vi "Teleop.vi"(10 "Match Info":T1={"Autonomous Elapsed Seconds"=0.0, "TeleOp Elapsed Seconds"=0.0, "Disabled Elapsed Seconds"=0.0, "Visited Autonomous"=FALSE, "Visited TeleOp"=FALSE, "Visited Disabled"=FALSE, "Autonomous Settings"={"Autonomous Style"=enum."Independent", "VI Refnum"=refnum}}, 11 "Call Context":T2) -> ()   [LabVIEW 2019]
doc: "This VI is called for each TeleOp packet received from the DS where the robot is not disabled. It is often used to read from the joysticks and update I/O or to update setpoints for timed control loops. It should complete and return within 20 milliseconds or it may miss DS packets."
uses:
  <vilib>/Rock Robotics/WPI/DriverStation/WPI_DriverStationDerivedRobotMode.ctl
  <vilib>/Rock Robotics/WPI/DriverStation/WPI_DriverStationMatch Info.ctl
  <vilib>/Rock Robotics/WPI/Utilities/WPI_GetSetVariantRefNum.vi
  <vilib>/Rock Robotics/Network Tables/NT Write Numeric Array.vi
  <vilib>/Rock Robotics/Network Tables/NT Read Boolean.vi
  <vilib>/Rock Robotics/Network Tables/NT Read Number.vi
  <vilib>/Rock Robotics/Network Tables/NT Write Boolean Array.vi
panel:
  in  "45 % DC":bool
  in  "35 % DC":bool
  in  "25 % DC":bool
  out "Sample Slider 0":dbl(slide) scale=0.0..5.0
  out "Sample Boolean 1":bool
  out "Sample Boolean 0":bool
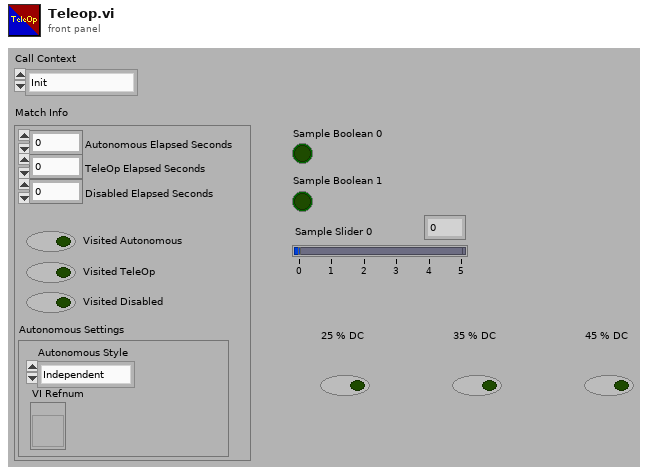
[diagram p1: front panel]
types:
  T1 = typedef "WPI_DriverStationMatch Info.ctl" = cluster{"Autonomous Elapsed Seconds":dbl, "TeleOp Elapsed Seconds":dbl, "Disabled Elapsed Seconds":dbl, "Visited Autonomous":bool, "Visited TeleOp":bool, "Visited Disabled":bool, "Autonomous Settings":cluster{"Autonomous Style":enum16{"Iterative", "Independent"}, "VI Refnum":refnum<vi>}}
  T2 = typedef "WPI_DriverStationDerivedRobotMode.ctl" = enum16{"Init", "Execute", "Stop"}
  T3 = typedef "WPI_JoystickDevRef.ctl" = cluster{"Device":T4}
  T4 = typedef "WPI_JoystickDeviceEnum.ctl" = enum16{"USB 0", "USB 1", "USB 2", "USB 3", "USB 4", "USB 5"}
  T5 = typedef "WPI_RobotDriveDevRef.ctl" = cluster{"DevStatus":errorcluster, "Motors[]":T6[], "Square Inputs":bool, "Max Output":dbl}
  T6 = typedef "WPI_MotorControlDeviceRef.ctl" = cluster{"DeviceStatus":errorcluster, "Type":T7, "PWM":cluster{"PWM Channel":T8, "DeadBand":T9}, "CAN":cluster{"Device Number":u8, "SetOutput VI Ref":variant, "GetOutput VI Ref":variant, "Enable VI Ref":variant, "Disable VI Ref":variant, "Data":variant}, "Invert":bool, "DIO PWM":cluster{"PWM \"Enable\" Channel":T8, "DIOChannel":T10, "PWM Rate":dbl}}
  T7 = typedef "WPI_MotorControlType.ctl" = enum16{"PWM", "CAN", "DIO PWM"}
  T8 = typedef "FPGA_DIOPWMChannel.ctl" = enum8{"PWM 0", "PWM 1", "PWM 2", "PWM 3", "PWM 4", "PWM 5", "PWM 6", "PWM 7", "PWM 8", "PWM 9", "PWM MXP 0", "PWM MXP 1", "PWM MXP 2", "PWM MXP 3", "PWM MXP 4", "PWM MXP 5", "PWM MXP 6", "PWM MXP 7", "PWM MXP 8", "PWM MXP 9", "Invalid"}
  T9 = typedef "WPI_PWMDeadband.ctl" = cluster{"Name":string, "maxPositivePwm":i32, "minPositivePwm":i32, "centerPwm":i32, "maxNegativePwm":i32, "minNegativePwm":i32, "angularRange":u16}
  T10 = typedef "FPGA_DIOChannel.ctl" = enum8{"DIO 0", "DIO 1", "DIO 2", "DIO 3", "DIO 4", "DIO 5", "DIO 6", "DIO 7", "DIO 8", "DIO 9", "DIO MXP 0", "DIO MXP 1", "DIO MXP 2", "DIO MXP 3", "DIO MXP 4", "DIO MXP 5", "DIO MXP 6", "DIO MXP 7", "DIO MXP 8", "DIO MXP 9", "DIO MXP 10", "DIO MXP 11", "DIO MXP 12", "DIO MXP 13", "DIO MXP 14", "DIO MXP 15", "SPI Port CS1", "SPI Port CS2", "SPI Port CS3", "SPI Port MISO", "SPI Port MOSI", "Invalid"}
  T11 = cluster{"JoystickDevRef":T3, "RobotDriveDevRef":T5}
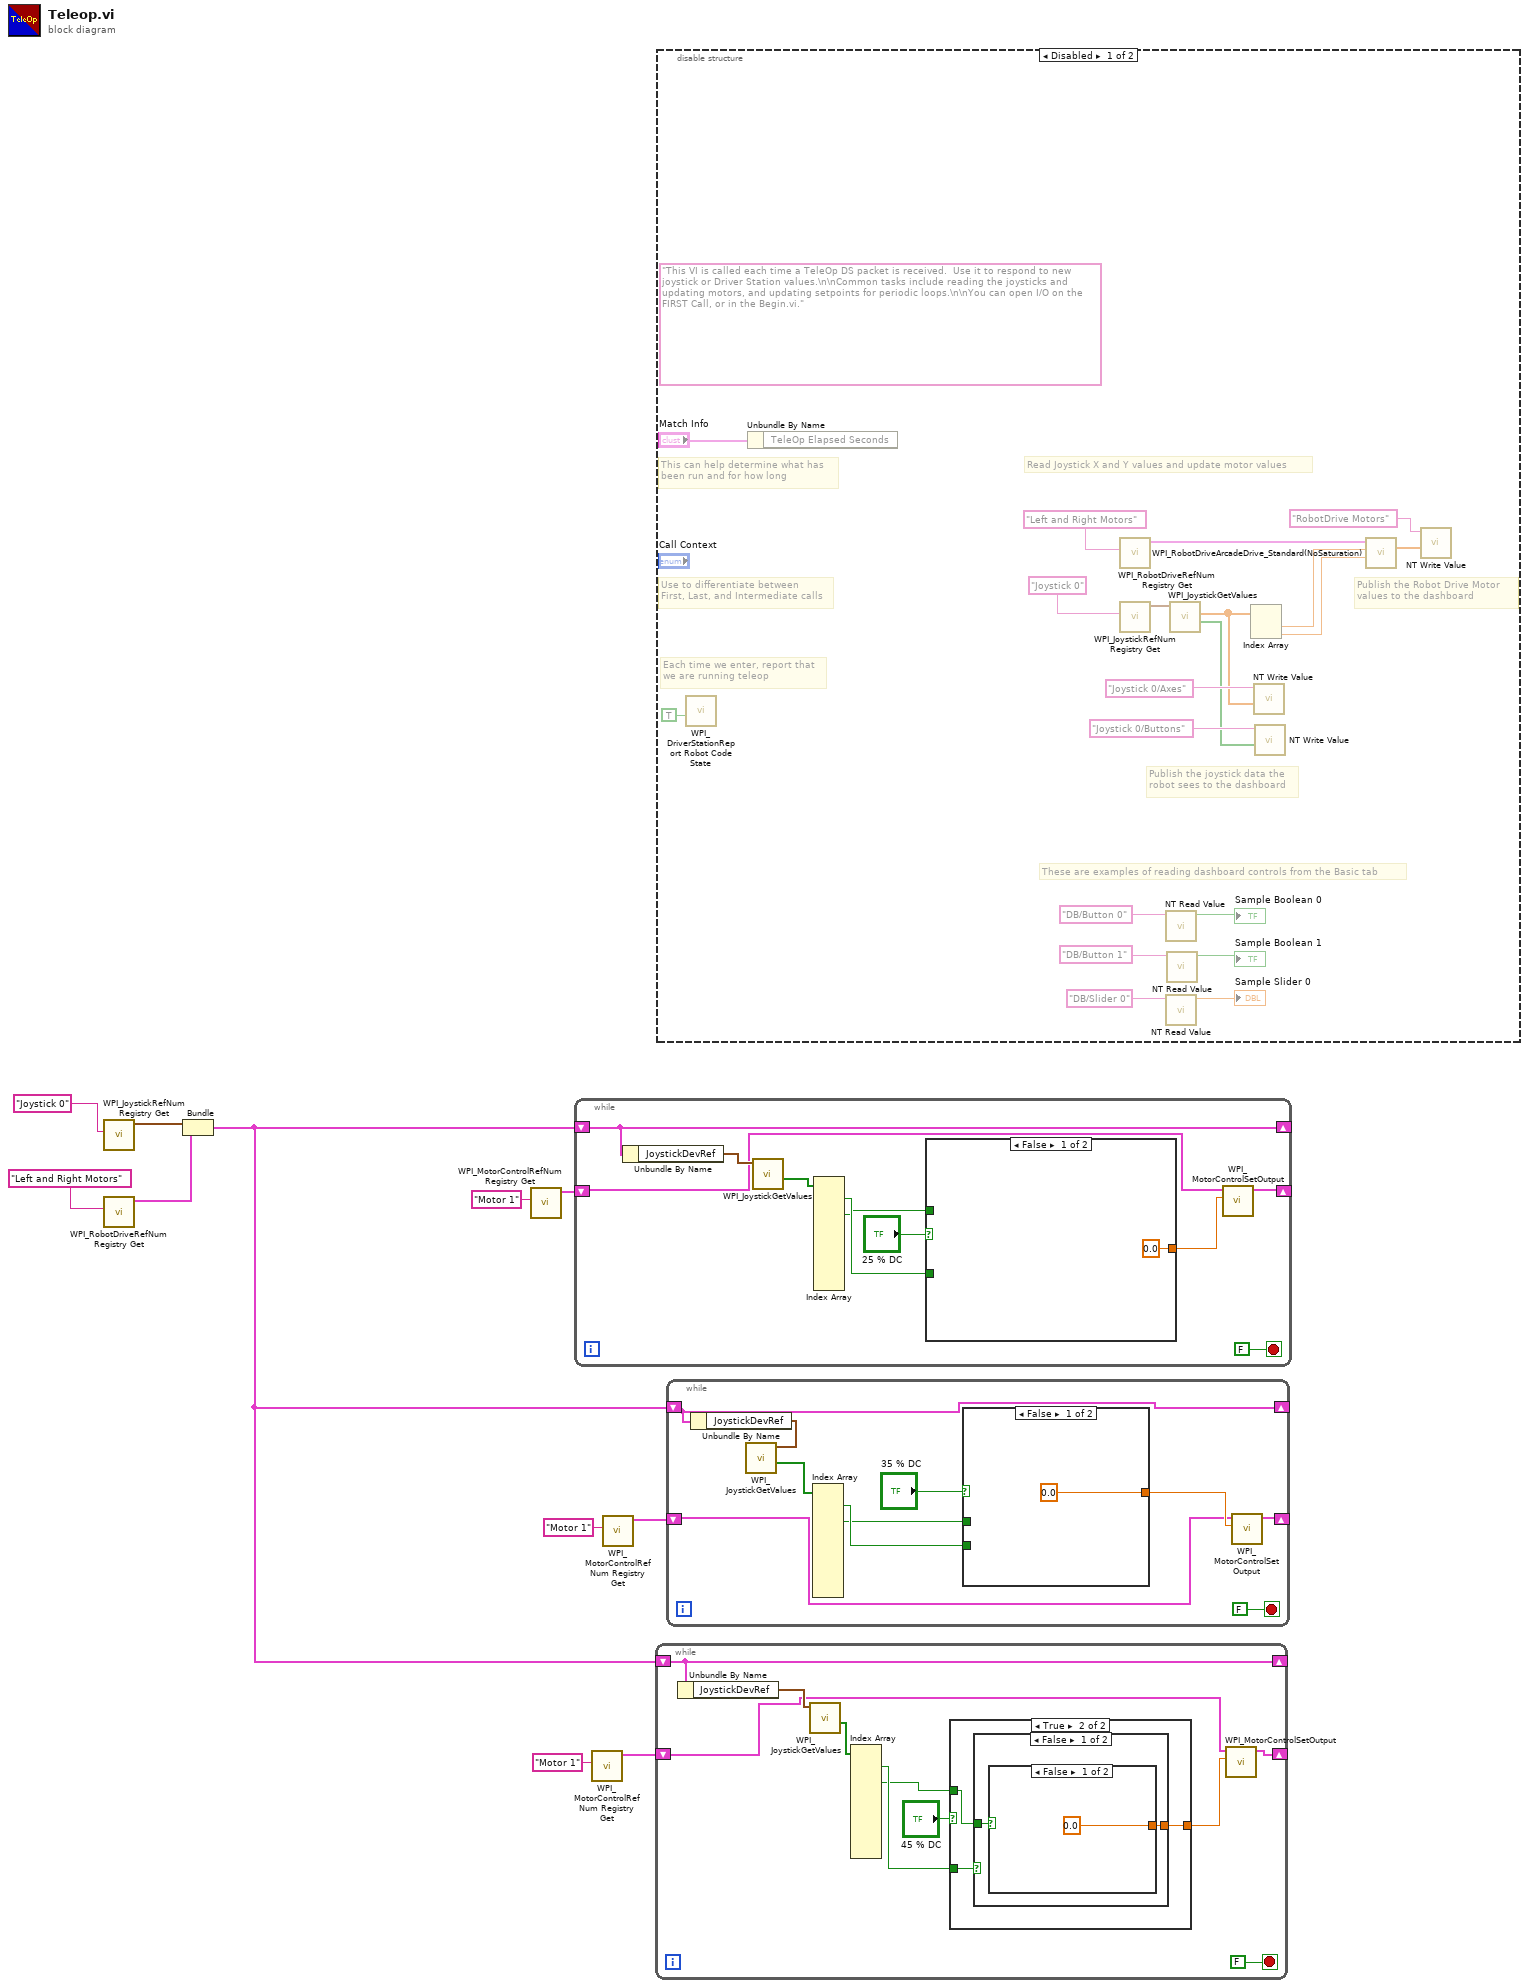
[diagram p0: block diagram]
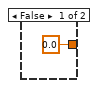
[diagram p2: hidden frame]
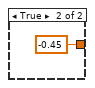
[diagram p3: hidden frame]
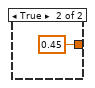
[diagram p4: hidden frame]
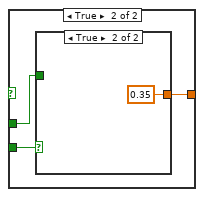
[diagram p5: hidden frame]
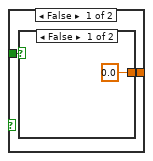
[diagram p6: hidden frame]
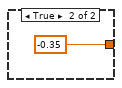
[diagram p7: hidden frame]
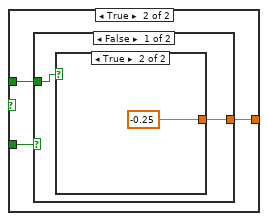
[diagram p8: hidden frame]
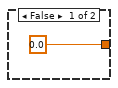
[diagram p9: hidden frame]
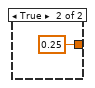
[diagram p10: hidden frame]
diagram:
  n1 = call <vilib>:"WPI_JoystickRefNum Registry Get.vi"("refnum name"="Joystick 0") -> ("JoystickDevRef"=w10:T3)  [unwired: 1 in, 9 out]
  n2 = call <vilib>:"WPI_RobotDriveRefNum Registry Get.vi"("refnum name"="Left and Right Motors") -> ("RobotDriveDevRef"=w9:T5)  [unwired: 1 in, 9 out]
  n3 = Bundle("JoystickDevRef"=w10, "RobotDriveDevRef"=w9) -> (w7:T11)  [unwired: 1 out]
  n4 = call <vilib>:"WPI_MotorControlRefNum Registry Get.vi"("refnum name"="Motor 1") -> ("MotorControlDevRef"=w6:T6)  [unwired: 9 in, 1 out]
  n5 = while {
    shift-right: [w19] -> _
    shift-left: w7 -> [w19]
    shift-right: [w16] -> _
    shift-left: w6 -> [w14]
    stop <- FALSE stop-if-true
    n6 = Unbundle By Name(w19) -> ("JoystickDevRef"=w18:T3)
    n7 = call <vilib>:"WPI_JoystickGetValues.vi"("JoystickDevRef"=w18) -> ("Buttons"=w17:bool[])  [unwired: 6 in, 4 out]
    n8 = Index Array(array=w17) -> (element #1=w13:bool, element #3=w12:bool)  [unwired: 12 in, 10 out]
    n9 = case shown="False" "25 % DC" {
      tunnel: [0.0 ("Output") w25] -> w15
      tunnel: w13 -> [_ w24]
      tunnel: w12 -> [_ w23]
      frame False {
      }
      frame True {
        n10 = case shown="False" w24 {
          tunnel: [w27 0.25 ("Output")] -> w25
          tunnel: w23 -> [w26 _]
          frame False {
            n11 = case shown="True" w26 {
              tunnel: [0.0 ("Output") -0.25 ("Output")] -> w27
              frame False {
              }
              frame True {
              }
            }
          }
          frame True {
          }
        }
      }
    }
    n12 = call <vilib>:"WPI_MotorControlSetOutput.vi"("Output"=w15, "MotorControlDevRef"=w14) -> ("MotorControlDevRef"=w16:T6)  [unwired: 7 in, 2 out]
  }
  n13 = call <vilib>:"WPI_MotorControlRefNum Registry Get.vi"("refnum name"="Motor 1") -> ("MotorControlDevRef"=w3:T6)  [unwired: 9 in, 1 out]
  n14 = call <vilib>:"WPI_MotorControlRefNum Registry Get.vi"("refnum name"="Motor 1") -> ("MotorControlDevRef"=w1:T6)  [unwired: 9 in, 1 out]
  n15 = while {
    shift-right: [w38] -> _
    shift-left: w7 -> [w38]
    shift-right: [w35] -> _
    shift-left: w3 -> [w33]
    stop <- FALSE stop-if-true
    n16 = Unbundle By Name(w38) -> ("JoystickDevRef"=w37:T3)
    n17 = call <vilib>:"WPI_JoystickGetValues.vi"("JoystickDevRef"=w37) -> ("Buttons"=w36:bool[])  [unwired: 6 in, 4 out]
    n18 = Index Array(array=w36) -> (element #1=w32:bool, element #3=w31:bool)  [unwired: 12 in, 10 out]
    n19 = case shown="True" "45 % DC" {
      tunnel: w32 -> [_ w44]
      tunnel: [0.0 ("Output") w43] -> w34
      tunnel: w31 -> [_ w42]
      frame False {
      }
      frame True {
        n20 = case shown="False" w44 {
          tunnel: [w46 0.45 ("Output")] -> w43
          tunnel: w42 -> [w45 _]
          frame False {
            n21 = case shown="False" w45 {
              tunnel: [0.0 ("Output") -0.45 ("Output")] -> w46
              frame False {
              }
              frame True {
              }
            }
          }
          frame True {
          }
        }
      }
    }
    n22 = call <vilib>:"WPI_MotorControlSetOutput.vi"("Output"=w34, "MotorControlDevRef"=w33) -> ("MotorControlDevRef"=w35:T6)  [unwired: 7 in, 2 out]
  }
  n23 = disable-structure shown="Disabled" {
    frame Disabled {
      (unwired) "This VI is called each time a TeleOp DS packet is received.  Use it to respond to new joystick or Driver Station values.\n\nCommon tasks include reading the joysticks and updating motors, and updating setpoints for periodic loops.\n\nYou can open I/O on the FIRST Call, or in the Begin.vi."
      # "These are examples of reading dashboard controls from the Basic tab"
      # "Publish the Robot Drive Motor\nvalues to the dashboard"
      # "Publish the joystick data the\nrobot sees to the dashboard"
      # "Each time we enter, report that\nwe are running teleop"
      # "Use to differentiate between\nFirst, Last, and Intermediate calls"
      # "This can help determine what has\nbeen run and for how long"
      # "Read Joystick X and Y values and update motor values"
      n24 = call <vilib>:"WPI_DriverStationReport Robot Code State.vi"("TeleOp"=TRUE ("Autonomous")) -> ()  [unwired: 10 in, 1 out]
      n25 = Unbundle By Name("Match Info") -> ()  [unwired: 1 out]
      n26 = call <vilib>:"WPI_RobotDriveRefNum Registry Get.vi"("refnum name"="Left and Right Motors") -> ("RobotDriveDevRef"=w67:T5)  [unwired: 1 in, 9 out]
      n27 = call <vilib>:"WPI_JoystickRefNum Registry Get.vi"("refnum name"="Joystick 0") -> ("JoystickDevRef"=w64:T3)  [unwired: 1 in, 9 out]
      n28 = call-poly <vilib>:"NT Read Value.vi"("Name"="DB/Button 0" ("refnum name")) -> ("Boolean"=→"Sample Boolean 0":bool)  [unwired: 9 in, 1 out]
      n29 = call-poly <vilib>:"NT Read Value.vi"("Name"="DB/Slider 0" ("refnum name")) -> ("Numeric"=→"Sample Slider 0":dbl)  [unwired: 9 in, 1 out]
      n30 = call-poly <vilib>:"NT Read Value.vi"("Name"="DB/Button 1" ("refnum name")) -> ("Boolean"=→"Sample Boolean 1":bool)  [unwired: 9 in, 1 out]
      n31 = call <vilib>:"WPI_JoystickGetValues.vi"("JoystickDevRef"=w64) -> ("Buttons"=w58:bool[], "Axes"=w59:dbl[])  [unwired: 6 in, 3 out]
      n32 = Index Array(array=w59) -> (element #1=w66:dbl, element #2=w62:dbl)  [unwired: 2 in]
      n33 = call-poly <vilib>:"NT Write Value.vi"("Numeric Array"=w59, "Name"="Joystick 0/Axes") -> ()  [unwired: 9 in, 1 out]
      n34 = call-poly <vilib>:"NT Write Value.vi"("Boolean Array"=w58, "Name"="Joystick 0/Buttons") -> ()  [unwired: 9 in, 1 out]
      n35 = call <vilib>:"WPI_RobotDriveArcadeDrive_Standard(NoSaturation).vi"("Y axis value"=w62, "X axis value"=w66, "RobotDriveDevRef"=w67) -> ("Motor Values"=w51:dbl[])  [unwired: 1 in, 7 out]
      n36 = call-poly <vilib>:"NT Write Value.vi"("Numeric Array"=w51, "Name"="RobotDrive Motors") -> ()  [unwired: 9 in, 1 out]
    }
    frame Enabled {
    }
  }
  n37 = while {
    shift-right: [w77] -> _
    shift-left: w7 -> [w77]
    shift-right: [w74] -> _
    shift-left: w1 -> [w72]
    stop <- FALSE stop-if-true
    n38 = Unbundle By Name(w77) -> ("JoystickDevRef"=w76:T3)
    n39 = call <vilib>:"WPI_JoystickGetValues.vi"("JoystickDevRef"=w76) -> ("Buttons"=w75:bool[])  [unwired: 6 in, 4 out]
    n40 = Index Array(array=w75) -> (element #1=w71:bool, element #3=w70:bool)  [unwired: 12 in, 10 out]
    n41 = case shown="False" "35 % DC" {
      tunnel: [0.0 ("Output") w83] -> w73
      tunnel: w71 -> [_ w82]
      tunnel: w70 -> [_ w81]
      frame False {
      }
      frame True {
        n42 = case shown="True" w82 {
          tunnel: [w85 0.35 ("Output")] -> w83
          tunnel: w81 -> [w84 _]
          frame False {
            n43 = case shown="False" w84 {
              tunnel: [0.0 ("Output") -0.35 ("Output")] -> w85
              frame False {
              }
              frame True {
              }
            }
          }
          frame True {
          }
        }
      }
    }
    n44 = call <vilib>:"WPI_MotorControlSetOutput.vi"("Output"=w73, "MotorControlDevRef"=w72) -> ("MotorControlDevRef"=w74:T6)  [unwired: 7 in, 2 out]
  }
